vi "Set LogFile_msTickTimer.vi"(8 "error in (no error)":errorcluster, 10 "LogFile_msTickTimer":path, 11 "DbgTimers in":refnum<class "DbgTimers.lvclass">) -> (0 "error out":errorcluster, 3 "DbgTimers out":refnum<class "DbgTimers.lvclass">)   [LabVIEW 2017, in "DbgTimers.lvclass"]
doc: "Developed by Kevin Thompson\nkevin@thompsonengineering.net\n\nCopyright 2018-2020\nThompson Engineering, LLC"
uses:
  DbgTimers.lvclass
  DbgTimers.lvclass/DbgTimers.ctl
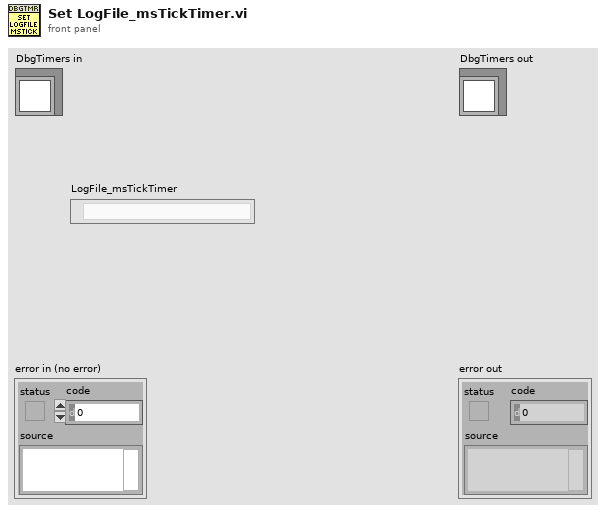
[diagram p1: front panel]
types:
  T1 = typedef "DbgTimers.lvclass/ObjData--cluster.ctl" = cluster{"Settings":T2, "ReadData-placeholder":T3, "Timers":T4, "Enable msTick Logging":bool, "LogFile_msTickTimer":path}
  T2 = typedef "DbgTimers.lvclass/Settings--cluster.ctl" = cluster{"Simulation":bool, "DbgTimer LogFolder":path}
  T3 = typedef "DbgTimers.lvclass/Read Data--cluster.ctl" = cluster{"Data":dbl}
  T4 = typedef "DbgTimers.lvclass/Timers--cluster.ctl" = cluster{"ms tick timers":T5[]}
  T5 = typedef "DbgTimers.lvclass/Millisecond Tick Timer--cluster.ctl" = cluster{"startTick":u32, "currentTick":u32, "elapsedTicks":u32, "totalElapsedTicks":u32}
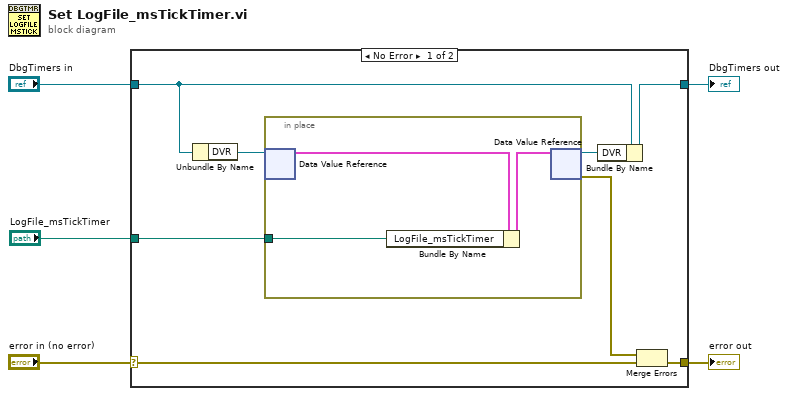
[diagram p0: block diagram]
diagram:
  n1 = case shown="No Error" "error in (no error)" {
    selector: "error in (no error)" -> [w13 w17]
    tunnel: [w7 w17] -> w4
    tunnel: [w9 w18] -> w2
    tunnel: "DbgTimers in" -> [w12 w18]
    tunnel: "LogFile_msTickTimer" -> [w8 _]
    frame No Error {
      n2 = Unbundle By Name(w12) -> ("DVR"=w11:refnum<data-value>)
      n3 = in-place {
        in-place-border: w8 -> [w14]
        n4 = in-place-dvr #1(w11) -> (w16:T1)  [unwired: 1 out]
        n5 = Bundle By Name(cluster=w16, "LogFile_msTickTimer"=w14) -> (w15:T1)
        n6 = in-place-dvr #1(w15) -> (w10:refnum<data-value>, w6:errorcluster)
      }
      n7 = Bundle By Name(cluster=w12, "DVR"=w10) -> (w9:refnum<class "DbgTimers.lvclass">)
      n8 = Merge Errors(w6, w13) -> (w7:errorcluster)
    }
    frame Error {
    }
  }
  "error out" <- w4
  "DbgTimers out" <- w2
